vi "FTW-Supervisor-CloseConnection.vi"(0 "FTW Supervisor Connection":refnum<class "FTW-Supervisor-Connector.lvclass">, 11 "error in":errorcluster) -> (15 "error out":errorcluster)   [LabVIEW 2014, in "FTW-Supervisor-Connector.lvclass"]
uses:
  FTW-Supervisor-Connector.lvclass
  FTW-Supervisor-Connector.lvclass/FTW-Supervisor-Connector.ctl
panel:
  # "Inputs"
  # "Outputs"
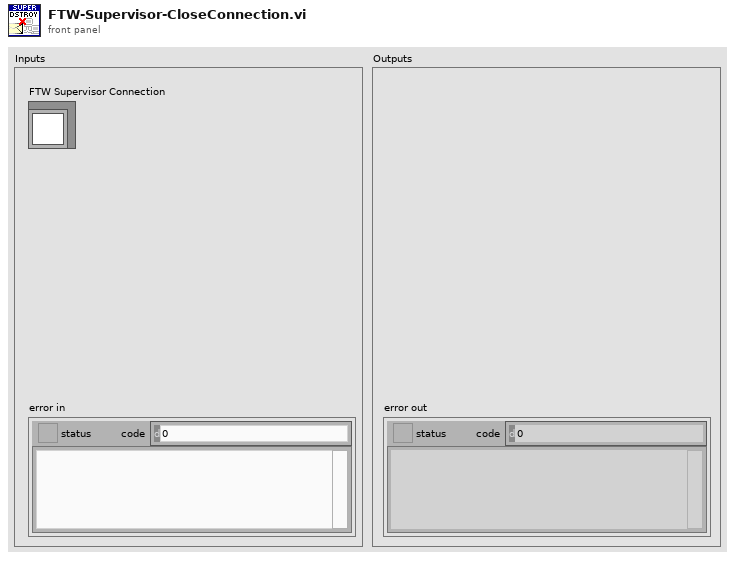
[diagram p1: front panel]
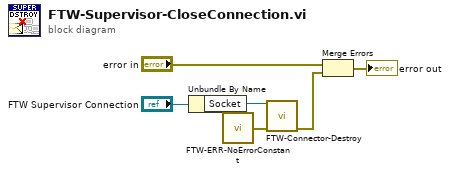
[diagram p0: block diagram]
diagram:
  n1 = Unbundle By Name("FTW Supervisor Connection") -> ("Socket"=w4:refnum<data-value>)
  n2 = call "FTW-ERR-NoErrorConstant.vi"() -> ("no error"=w2:errorcluster)
  n3 = call "FTW-Connector-Destroy.vi"("FTW Connector"=w4, "error in"=w2) -> ("error out"=w1:errorcluster)  [unwired: 13 in]
  n4 = Merge Errors("error in", w1) -> (→"error out":errorcluster)
